vi "Message Box.vi"(8 "Combo box values":string[](array[string]), 9 "On-Screen Keyboard Visible?":bool, 10 "Message":string, 11 "Type":u16(ring) items=["Information box", "Yes/No Prompt", "Value prompt", "Drop Down"]) -> (1 "Input String":string, 2 "Cancel":bool, 3 "Ok":bool)   [LabVIEW 2020]
uses:
  <vilib>/Utility/sysdir.llb/System Directory Type.ctl
panel:
  in  "Combo Box":string(combo)
  in  "Keyboard":bool
  in  "String Input":string
  in  "Cancel Button":bool
  in  "OK Button":bool
  # "Select the Direction"
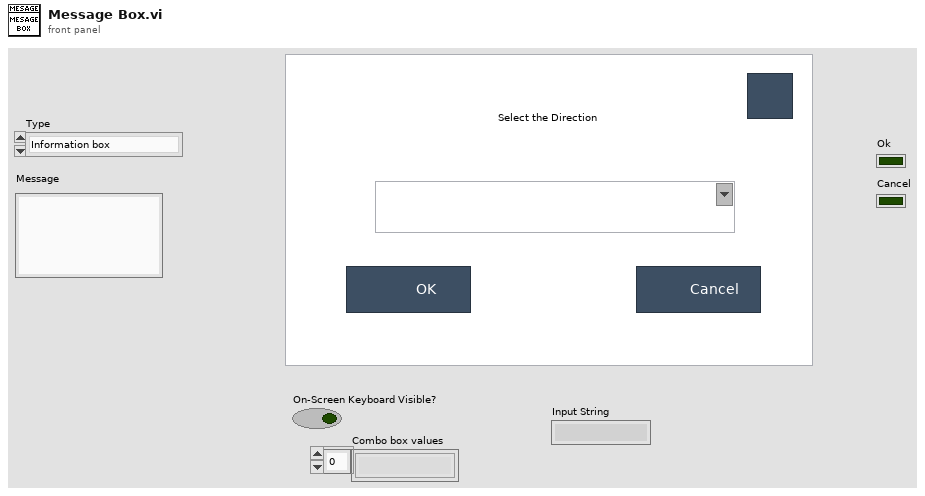
[diagram p1: front panel]
types:
  T1 = typedef "System Directory Type.ctl" = i32
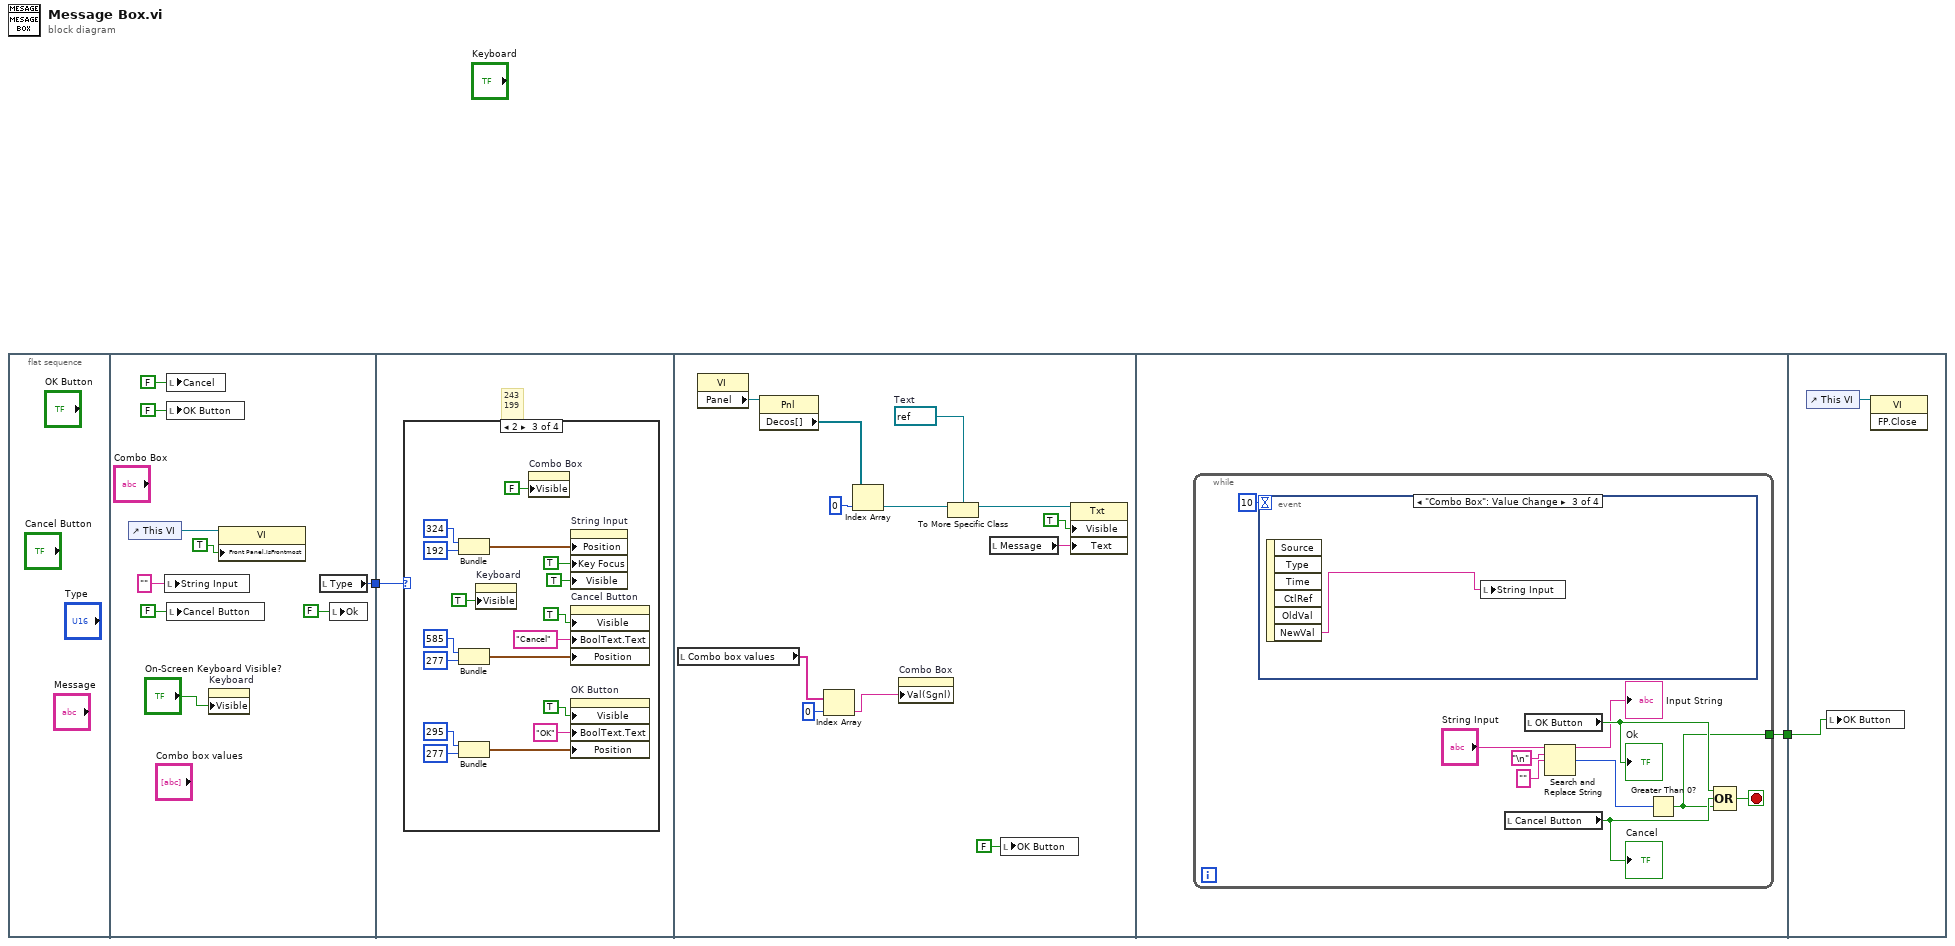
[diagram p0: block diagram]
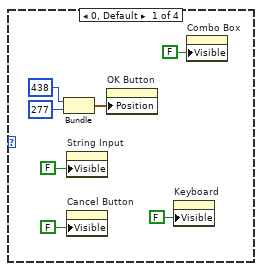
[diagram p2: hidden frame]
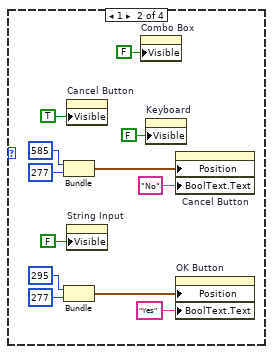
[diagram p3: hidden frame]
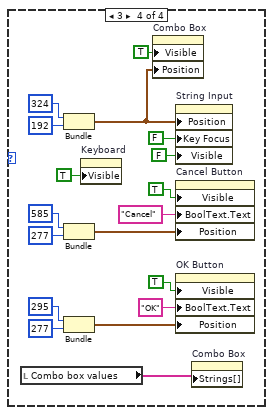
[diagram p4: hidden frame]
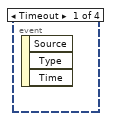
[diagram p5: hidden frame]
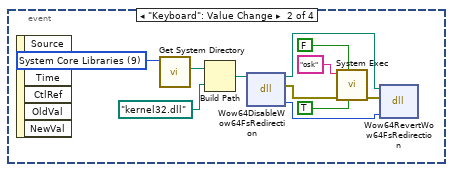
[diagram p6: hidden frame]
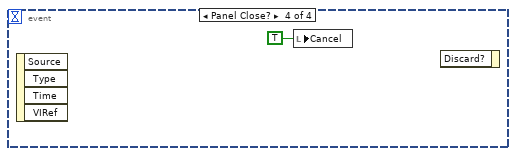
[diagram p7: hidden frame]
diagram:
  n1 = flat-sequence {
    tunnel: [w11] -> w2
    tunnel: w2 -> [w12]
    tunnel: [w79] -> w1
    tunnel: w1 -> [w103]
    frame #0 {
    }
    frame #1 {
      n2 = control-ref of="This VI"() -> (w6:refnum<vi>)
      n3 = local write "String Input"("" ("String Input")) -> ()
      n4 = local write "Cancel"(FALSE ("Cancel")) -> ()
      n5 = local write "OK Button"(FALSE ("OK Button")) -> ()
      n6 = local write "Cancel Button"(FALSE ("OK Button")) -> ()
      n7 = property on="Keyboard" class="Bool"("Visible"="On-Screen Keyboard Visible?") -> ()  [unwired: 2 in, 2 out]
      n8 = property class="VI"(reference=w6, "Front Panel.IsFrontmost"=TRUE ("Front Panel Window:Is Frontmost")) -> ()  [unwired: 1 in, 2 out]
      n9 = local read "Type"() -> (w11:u16)
      n10 = local write "Ok"(FALSE ("Ok")) -> ()
    }
    frame #2 {
      # "243\n199"
      n11 = case shown="2" w12 {
        frame 0, Default {
          n12 = Bundle(438, 277) -> (w17:cluster{i32, i32})  [unwired: 1 in]
          n13 = property on="String Input" class="Str"("Visible"=FALSE) -> ()  [unwired: 2 in, 2 out]
          n14 = property on="Cancel Button" class="Bool (strict)"("Visible"=FALSE) -> ()  [unwired: 2 in, 2 out]
          n15 = property on="OK Button" class="Bool (strict)"("Position"=w17) -> ()  [unwired: 2 in, 2 out]
          n16 = property on="Keyboard" class="Bool"("Visible"=FALSE) -> ()  [unwired: 2 in, 2 out]
          n17 = property on="Combo Box" class="CmbBox"("Visible"=FALSE) -> ()  [unwired: 2 in, 2 out]
        }
        frame 1 {
          n18 = Bundle(585, 277) -> (w27:cluster{i32, i32})  [unwired: 1 in]
          n19 = Bundle(295, 277) -> (w26:cluster{i32, i32})  [unwired: 1 in]
          n20 = property on="Cancel Button" class="Bool (strict)"("Visible"=TRUE) -> ()  [unwired: 2 in, 2 out]
          n21 = property on="String Input" class="Str"("Visible"=FALSE) -> ()  [unwired: 2 in, 2 out]
          n22 = property on="Combo Box" class="CmbBox"("Visible"=FALSE) -> ()  [unwired: 2 in, 2 out]
          n23 = property on="Keyboard" class="Bool"("Visible"=FALSE) -> ()  [unwired: 2 in, 2 out]
          n24 = property on="Cancel Button" class="Bool (strict)"("Position"=w27, "BoolText.Text"="No" ("Boolean Text.Text")) -> ()  [unwired: 2 in, 2 out]
          n25 = property on="OK Button" class="Bool (strict)"("Position"=w26, "BoolText.Text"="Yes" ("Boolean Text.Text")) -> ()  [unwired: 2 in, 2 out]
        }
        frame 2 {
          n26 = Bundle(324, 192) -> (w45:cluster{i32, i32})  [unwired: 1 in]
          n27 = Bundle(585, 277) -> (w35:cluster{i32, i32})  [unwired: 1 in]
          n28 = Bundle(295, 277) -> (w38:cluster{i32, i32})  [unwired: 1 in]
          n29 = property on="Keyboard" class="Bool"("Visible"=TRUE) -> ()  [unwired: 2 in, 2 out]
          n30 = property on="Combo Box" class="CmbBox"("Visible"=FALSE) -> ()  [unwired: 2 in, 2 out]
          n31 = property on="String Input" class="Str"("Position"=w45, "Key Focus"=TRUE, "Visible"=TRUE) -> ()  [unwired: 2 in, 2 out]
          n32 = property on="Cancel Button" class="Bool (strict)"("Visible"=TRUE, "BoolText.Text"="Cancel" ("Boolean Text.Text"), "Position"=w35) -> ()  [unwired: 2 in, 2 out]
          n33 = property on="OK Button" class="Bool (strict)"("Visible"=TRUE, "BoolText.Text"="OK" ("Boolean Text.Text"), "Position"=w38) -> ()  [unwired: 2 in, 2 out]
        }
        frame 3 {
          n34 = local read "Combo box values"() -> (w49:string[])
          n35 = Bundle(324, 192) -> (w50:cluster{i32, i32})  [unwired: 1 in]
          n36 = Bundle(585, 277) -> (w54:cluster{i32, i32})  [unwired: 1 in]
          n37 = Bundle(295, 277) -> (w57:cluster{i32, i32})  [unwired: 1 in]
          n38 = property on="Keyboard" class="Bool"("Visible"=TRUE) -> ()  [unwired: 2 in, 2 out]
          n39 = property on="Combo Box" class="CmbBox"("Visible"=TRUE, "Position"=w50) -> ()  [unwired: 2 in, 2 out]
          n40 = property on="String Input" class="Str"("Position"=w50, "Key Focus"=FALSE, "Visible"=FALSE) -> ()  [unwired: 2 in, 2 out]
          n41 = property on="Cancel Button" class="Bool (strict)"("Visible"=TRUE, "BoolText.Text"="Cancel" ("Boolean Text.Text"), "Position"=w54) -> ()  [unwired: 2 in, 2 out]
          n42 = property on="OK Button" class="Bool (strict)"("Visible"=TRUE, "BoolText.Text"="OK" ("Boolean Text.Text"), "Position"=w57) -> ()  [unwired: 2 in, 2 out]
          n43 = property on="Combo Box" class="CmbBox"("Strings[]"=w49) -> ()  [unwired: 2 in, 2 out]
        }
      }
    }
    frame #3 {
      w73 = refnum<vi> refnum  # Text
      n44 = local read "Combo box values"() -> (w69:string[])
      n45 = property class="VI"() -> ("Panel"=w76:refnum<vi>)  [unwired: 2 in, 2 out]
      n46 = property class="Pnl"(reference=w76) -> ("Decos[]"=w75:refnum<vi>[])  [unwired: 1 in, 2 out]
      n47 = Index Array(array=w69, index=0) -> (element=w67:string)
      n48 = Index Array(array=w75, index=0 ("index 2")) -> (element=w77:refnum<vi>)
      n49 = property on="Combo Box" class="CmbBox"("Val(Sgnl)"=w67) -> ()  [unwired: 2 in, 2 out]
      n50 = To More Specific Class(target class=w73, reference=w77) -> (specific class reference=w78:refnum<vi>)  [unwired: 1 in, 1 out]
      n51 = local read "Message"() -> (w71:string)
      n52 = local write "OK Button"(FALSE ("OK Button")) -> ()
      n53 = property class="Txt"(reference=w78, "Visible"=TRUE, "Text"=w71) -> ()  [unwired: 1 in, 2 out]
    }
    frame #4 {
      n54 = while {
        tunnel: [w80] -> w79
        stop <- w88 stop-if-true
        n55 = event shown="[2] \"Combo Box\": Value Change" {
          selector: _ -> [_ _ _ _]
          dyn-events: _ -> [_ _ _ _]
          timeout: 10 -> [_ _ _ _]
          event Timeout {
            n56 = event-data() -> ()  [unwired: 1 in, 3 out]
          }
          event "Keyboard": Value Change {
            w96 = T1 9 items=["User Home"=0, "User Desktop"=1, "User Documents"=2, "User Application Data"=3, "User Preferences"=4, "User Temporary"=5, "Public Documents"=6, "Public Application Data"=7, "Public Preferences"=8, "Public Cache"=13, "System Core Libraries"=9, "System Installed Libraries"=10, "Application Files"=11, "Boot Volume Root"=12] ("system directory type")
            n57 = event-data() -> ()  [unwired: 1 in, 6 out]
            n58 = call <vilib>:"Get System Directory.vi"("system directory type"=w96) -> ("system directory"=w99:path)  [unwired: 10 in]
            n59 = Build Path(base path=w99, name or relative path=path "kernel32.dll") -> (appended path=w98:path)
            n60 = dll-call lib="C:/Windows/System32/kernel32.dll" fn="Wow64DisableWow64FsRedirection"(path in=w98) -> (path out=w100:path, error out=w95:errorcluster, "arg1"=w91:i32)  [unwired: 4 in]
            n61 = call <vilib>:"System Exec.vi"("run minimized? (F)"=TRUE, "wait until completion? (T)"=FALSE, "error in (no error)"=w95, "command line"="osk") -> ("error out"=w94:errorcluster)  [unwired: 4 in, 3 out]
            n62 = dll-call lib="C:/Windows/System32/kernel32.dll" fn="Wow64RevertWow64FsRedirection"(path in=w100, error in=w94, "arg1"=w91) -> ()  [unwired: 3 in, 2 out]
          }
          event "Combo Box": Value Change {
            n63 = event-data() -> ("NewVal"=w101:string)  [unwired: 1 in, 5 out]
            n64 = local write "String Input"(w101) -> ()
          }
          event Panel Close? {
            n65 = event-data() -> ()  [unwired: 1 in, 4 out]
            n66 = local write "Cancel"(TRUE ("Cancel")) -> ()
            n67 = event-data() -> ()  [unwired: 2 in, 1 out]
          }
        }
        n68 = local read "Cancel Button"() -> (w87:bool)
        "Cancel" <- w87
        n69 = local read "OK Button"() -> (w89:bool)
        "Ok" <- w89
        n70 = Search and Replace String(input string="String Input", search string="\n", replace string="" ("replace string (\"\")")) -> (result string=→"Input String":string, number of replacements=w83:i32)  [unwired: 5 in, 2 out]
        n71 = Greater Than 0?(x=w83) -> (x > 0?=w80:bool)
        n72 = Compound Arithmetic op=OR(w89, w87, w80) -> (w88:bool)
      }
    }
    frame #5 {
      n73 = control-ref of="This VI"() -> (w104:refnum<vi>)
      n74 = local write "OK Button"(w103) -> ()
      n75 = invoke class="VI" method="FP.Close"(reference=w104) -> ()  [unwired: 2 in, 3 out]
    }
  }
